vi "communicate.vi"(0 "Communication in":refnum<class "Communication.lvclass">, 1 "grSIM replacement":cluster{"robots":T4[], "ball":T5}, 2 "replace active":bool, 5 "Game":refnum<class "Game.lvclass">, 7 "Com UDP":T3={"UDP GrSim TX"=TRUE, "Address:"="127.0.0.1", "Port:"=20011}, 9 "Com Serial":T2, 11 "error in (no error)":errorcluster, 12 "Com SOS":T1={"UDP SOS TX "=FALSE, "SOS Port: 2"=10025, "SOS Port: "=10021, "SOS Address:"="192.168.0.101"}, 13 "FIRASim?":bool=TRUE) -> (4 "Communication out":refnum<class "Communication.lvclass">, 6 "Comm TX FPS":dbl, 10 "AllyRef":refnum<class "Ally.lvclass">, 15 "error out":errorcluster)   [LabVIEW 2023, in "Communication.lvclass"]
uses:
  Communication.lvclass
  Paths/grSim Packet Command UDP Test Folder/grSim/grSim RobotReplacement.ctl
  Paths/grSim Packet Command UDP Test Folder/grSim/grSim_BallReplacement.ctl
  Vision_class/Old vision/SSL Detection Frame Simple Estimator Cameras VelCmd Folder/Core/AI Input.ctl
  Vision_class/Old vision/Controls/AI Robot.ctl
  Vision_class/Old vision/Controls/Functions Enum.ctl
  Vision_class/Old vision/Controls/AttackerStates.ctl
  Vision_class/Old vision/Controls/PathDests.ctl
  Vision_class/Old vision/Controls/PathDest.ctl
  Game_class/Navigation/VSSNavigation/VSSAttackerStates.ctl
  Vision_class/Old vision/SSL Detection Frame Simple Estimator Cameras VelCmd Folder/Core/AI Ball.ctl
  Vision_class/Old vision/SSL Detection Frame Simple Estimator Cameras VelCmd Folder/Core/Field Size.ctl
  Vision_class/Old vision/SSL Detection Frame Simple Estimator Cameras VelCmd Folder/Core/AI Judge.ctl
  Paths/MessageAI_State Folder/Intel/Command Enum.ctl
  Vision_class/Old vision/SSL Detection Frame Simple Estimator Cameras VelCmd Folder/Util/Events/Events.ctl
  Game_class/Game.lvclass
  Controls/ComUDP.ctl
  Controls/ComSerial.ctl
  Controls/ComSOS.ctl
  Ally_class/Ally.lvclass
panel:
  in  "IA States":T6={"our_robots"=[], "enemy_robots"=[], "balls"=[], "geometry"={"line_width"=0, "field_length"=0, "field_width"=0, "boundary_width"=0, "referee_width"=0, "goal_width"=0, "goal_depth"=0, "goal_wall_width"=0, "center_circle_radius"=0, "defense_radius"=0, "defense_stretch"=0, "free_kick_from_defense_dist"=0, "penalty_spot_from_field_line_dist"=0, "penalty_line_from_spot_dist"=0}, "IA Judge"={"stage"="", "command"="", "our_goalie_id"=0.0, "enemy_goalie_id"=0.0, "command enum"=enum."Halt", "Time"=enum."Azul"}, "Received Timestamp"=timestamp(0 s since 1904-01-01), "Events"={"Touch"=FALSE, "Ball out"=FALSE, "id touch"=0.0, "Ball out of \nVision"=FALSE, "Ball inside \nGoalie area"=FALSE, "Robot not responding"=FALSE, "Robots responding status"=[1.0, 1.0, 1.0, 1.0, 1.0, 1.0], "Enemy Ball \nPossession"=FALSE, "Pass State"=FALSE, "id end of pass"=0.0, "Kick"=FALSE, "Id ini Possession"=0.0, "Ball Possesion"=FALSE, "Id Possesion"=0.0, "Direct Kick"=FALSE, "2nd Strk Ativo"=FALSE}}
  out "grSim":cluster{"robots":T4[], "ball":T5}
  out "Total Delay":dbl format="%#.5g"
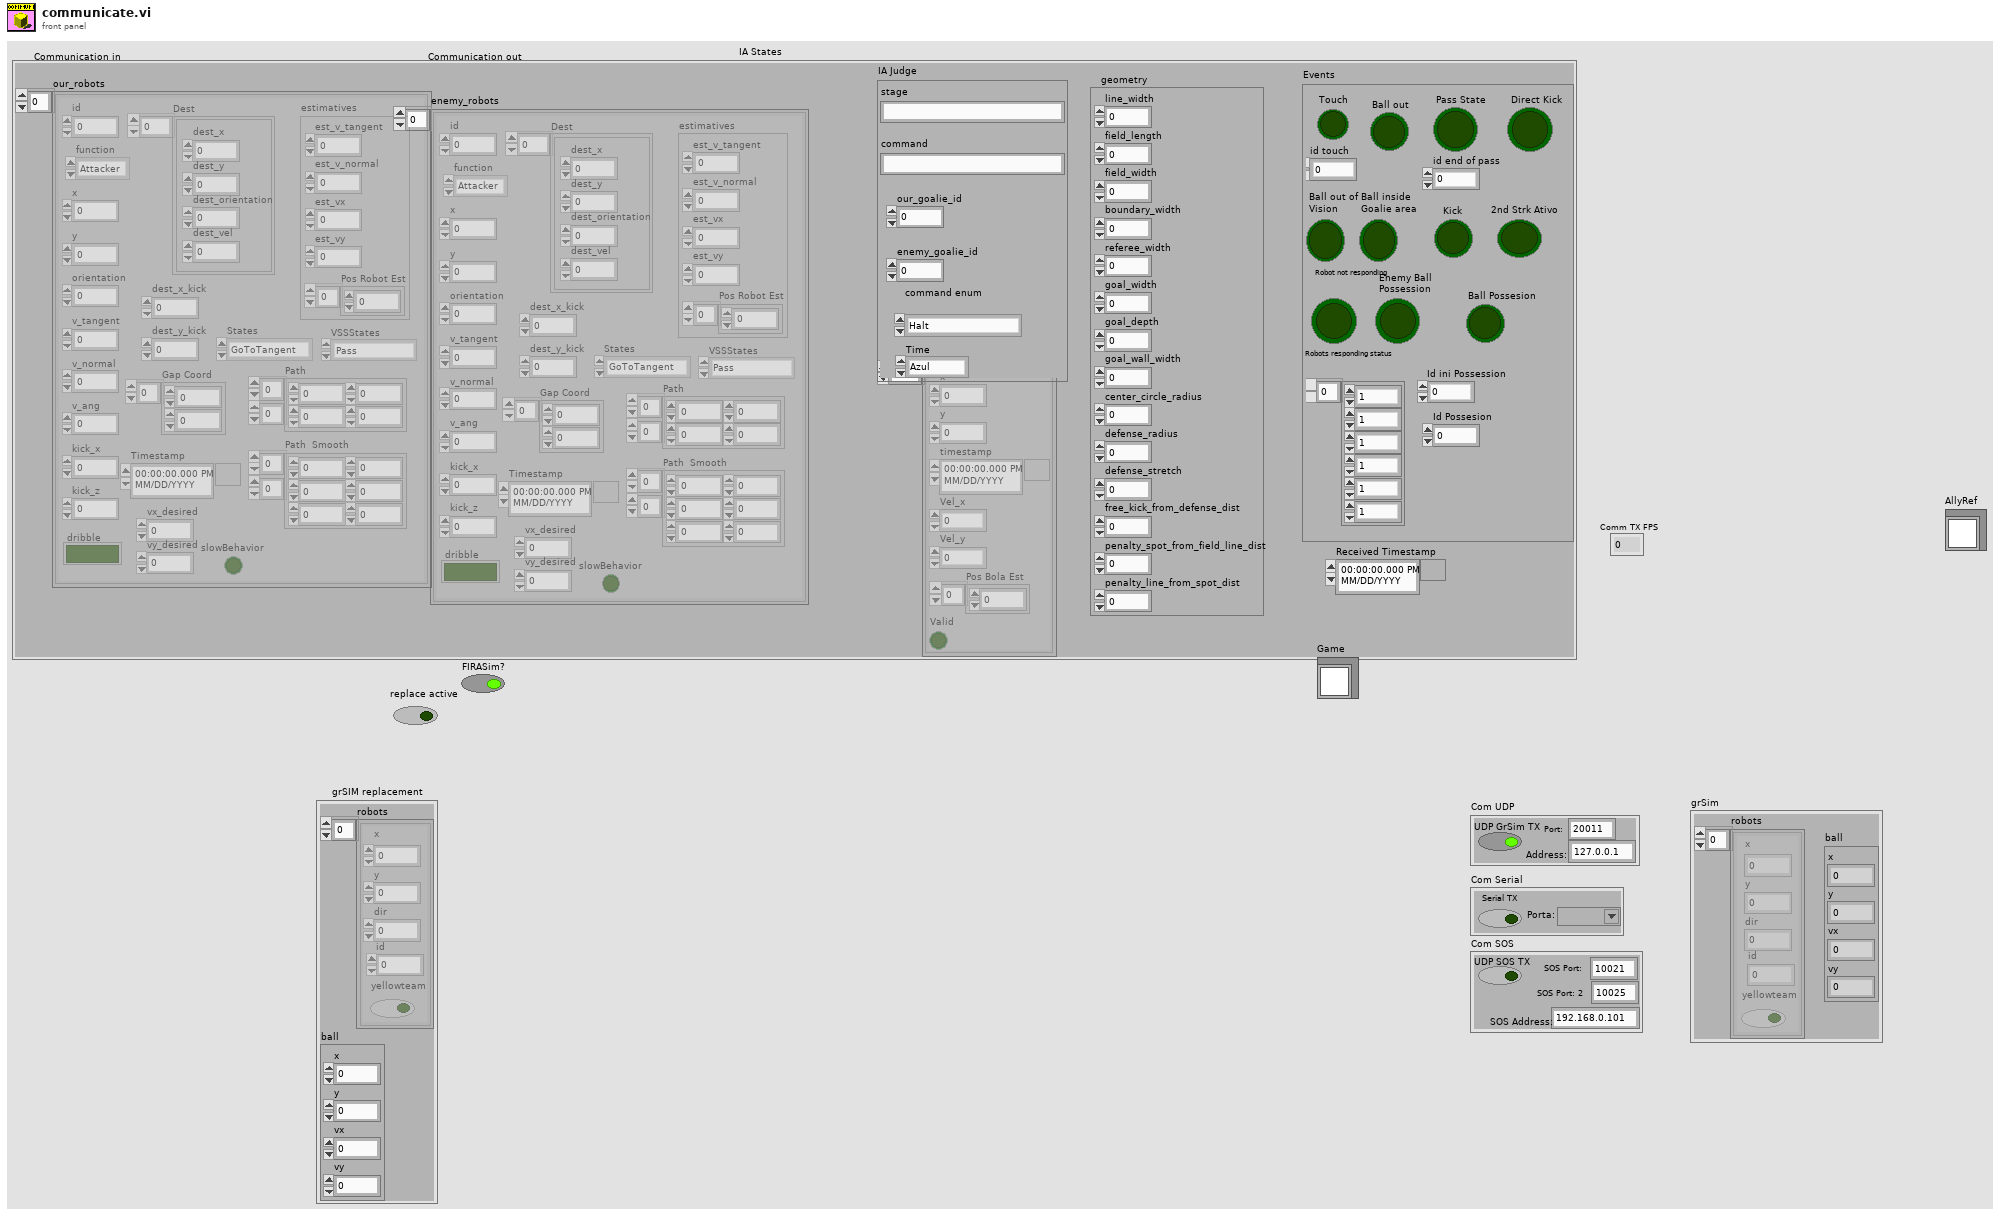
[diagram p1: front panel]
types:
  T1 = typedef "ComSOS.ctl" = cluster{"UDP SOS TX ":bool, "SOS Port: 2":u16, "SOS Port: ":u16, "SOS Address:":string}
  T2 = typedef "ComSerial.ctl" = cluster{"Serial TX":bool, "Porta:":refnum<visa-resource-name>}
  T3 = typedef "ComUDP.ctl" = cluster{"UDP GrSim TX":bool, "Address:":string, "Port:":u16}
  T4 = typedef "grSim RobotReplacement.ctl" = cluster{"x":dbl, "y":dbl, "dir":dbl, "yellowteam":bool, "id":u32}
  T5 = typedef "grSim_BallReplacement.ctl" = cluster{"x":dbl, "y":dbl, "vx":dbl, "vy":dbl}
  T6 = typedef "AI Input.ctl" = cluster{"our_robots":T7[], "enemy_robots":T7[], "balls":T13[], "geometry":T14, "IA Judge":T15, "Received Timestamp":timestamp, "Events":T17}
  T7 = typedef "AI Robot.ctl" = cluster{"id":u32, "function":T8, "x":dbl, "y":dbl, "orientation":dbl, "v_tangent":dbl, "v_normal":dbl, "v_ang":dbl, "kick_x":dbl, "kick_z":dbl, "dribble":bool, "Timestamp":timestamp, "estimatives":cluster{"est_v_tangent":dbl, "est_v_normal":dbl, "est_vx":dbl, "est_vy":dbl, "Pos Robot Est":dbl[]}, "dest_x_kick":dbl, "dest_y_kick":dbl, "Gap Coord":dbl[], "States":T9, "Path ":dbl[][], "Path  Smooth":dbl[][], "Dest":T10, "vx_desired":dbl, "vy_desired":dbl, "slowBehavior":bool, "VSSStates":T12}
  T8 = typedef "Functions Enum.ctl" = enum16{"2nd Striker", "Attacker", "Goalie", "Defender", "Striker", "Goto 0", "Dummy", "Kicker", "ZigZag 0", "ZigZag 1", "ZigZag 2", "ZigZag 3", "ZigZag 4", "ZigZag 5", "ZigZag 6", "ZigZag 7", "ZigZag 8", ""}
  T9 = typedef "AttackerStates.ctl" = enum16{"Pass", "GoToTangent", "BallGetting", "GoToKick", ""}
  T10 = typedef "PathDests.ctl" = T11[]
  T11 = typedef "PathDest.ctl" = cluster{"dest_x":dbl, "dest_y":dbl, "dest_orientation":dbl, "dest_vel":dbl}
  T12 = typedef "VSSAttackerStates.ctl" = enum16{"Pass", "GoToTangent", "BallGetting", "GoToKick", "Rotate anti-clockwise", "Rotate Clockwise", ""}
  T13 = typedef "AI Ball.ctl" = cluster{"x":dbl, "y":dbl, "timestamp":timestamp, "Vel_x":dbl, "Vel_y":dbl, "Pos Bola Est":dbl[], "Valid":bool}
  T14 = typedef "Field Size.ctl" = cluster{"line_width":u32, "field_length":u32, "field_width":u32, "boundary_width":u32, "referee_width":u32, "goal_width":u32, "goal_depth":u32, "goal_wall_width":u32, "center_circle_radius":u32, "defense_radius":u32, "defense_stretch":u32, "free_kick_from_defense_dist":u32, "penalty_spot_from_field_line_dist":u32, "penalty_line_from_spot_dist":u32}
  T15 = typedef "AI Judge.ctl" = cluster{"stage":string, "command":string, "our_goalie_id":dbl, "enemy_goalie_id":dbl, "command enum":T16, "Time":enum16{"Azul", "Amarelo"}}
  T16 = typedef "Command Enum.ctl" = enum16{"Halt", "Stop", "Force Start", "PKA Normal Start", "Prepare Kickoff Ally", "PKE Normal Start", "Prepare Kickoff Enemy", "Prepare Penalty Ally", "PPA Normal Start", "Prepare Penalty Enemy", "PPE Normal Start", "Direct Free Enemy", "Direct Free Ally", "Indirect Free Enemy", "Indirect Free Ally", "Timeout Enemy", "Timeout Ally", "Goal Enemy", "Goal Ally", "Ball Placement Enemy", "Ball Placement Ally", "Normal Half Time", "Extra Time Break", "Extra Half Time", "None", "Post Game"}
  T17 = typedef "Events.ctl" = cluster{"Touch":bool, "Ball out":bool, "id touch":dbl, "Ball out of \nVision":bool, "Ball inside \nGoalie area":bool, "Robot not responding":bool, "Robots responding status":dbl[], "Enemy Ball \nPossession":bool, "Pass State":bool, "id end of pass":dbl, "Kick":bool, "Id ini Possession":dbl, "Ball Possesion":bool, "Id Possesion":dbl, "Direct Kick":bool, "2nd Strk Ativo":bool}
  T18 = typedef "grSim Robot Command.ctl" = cluster{"id":u32, "kickspeedx":sgl, "kickspeedz":sgl, "veltangent":sgl, "velnormal":sgl, "velangular":sgl, "spinner":bool, "wheelspeed":bool, "wheel1":sgl, "wheel2":sgl, "wheel3":sgl, "wheel4":sgl}
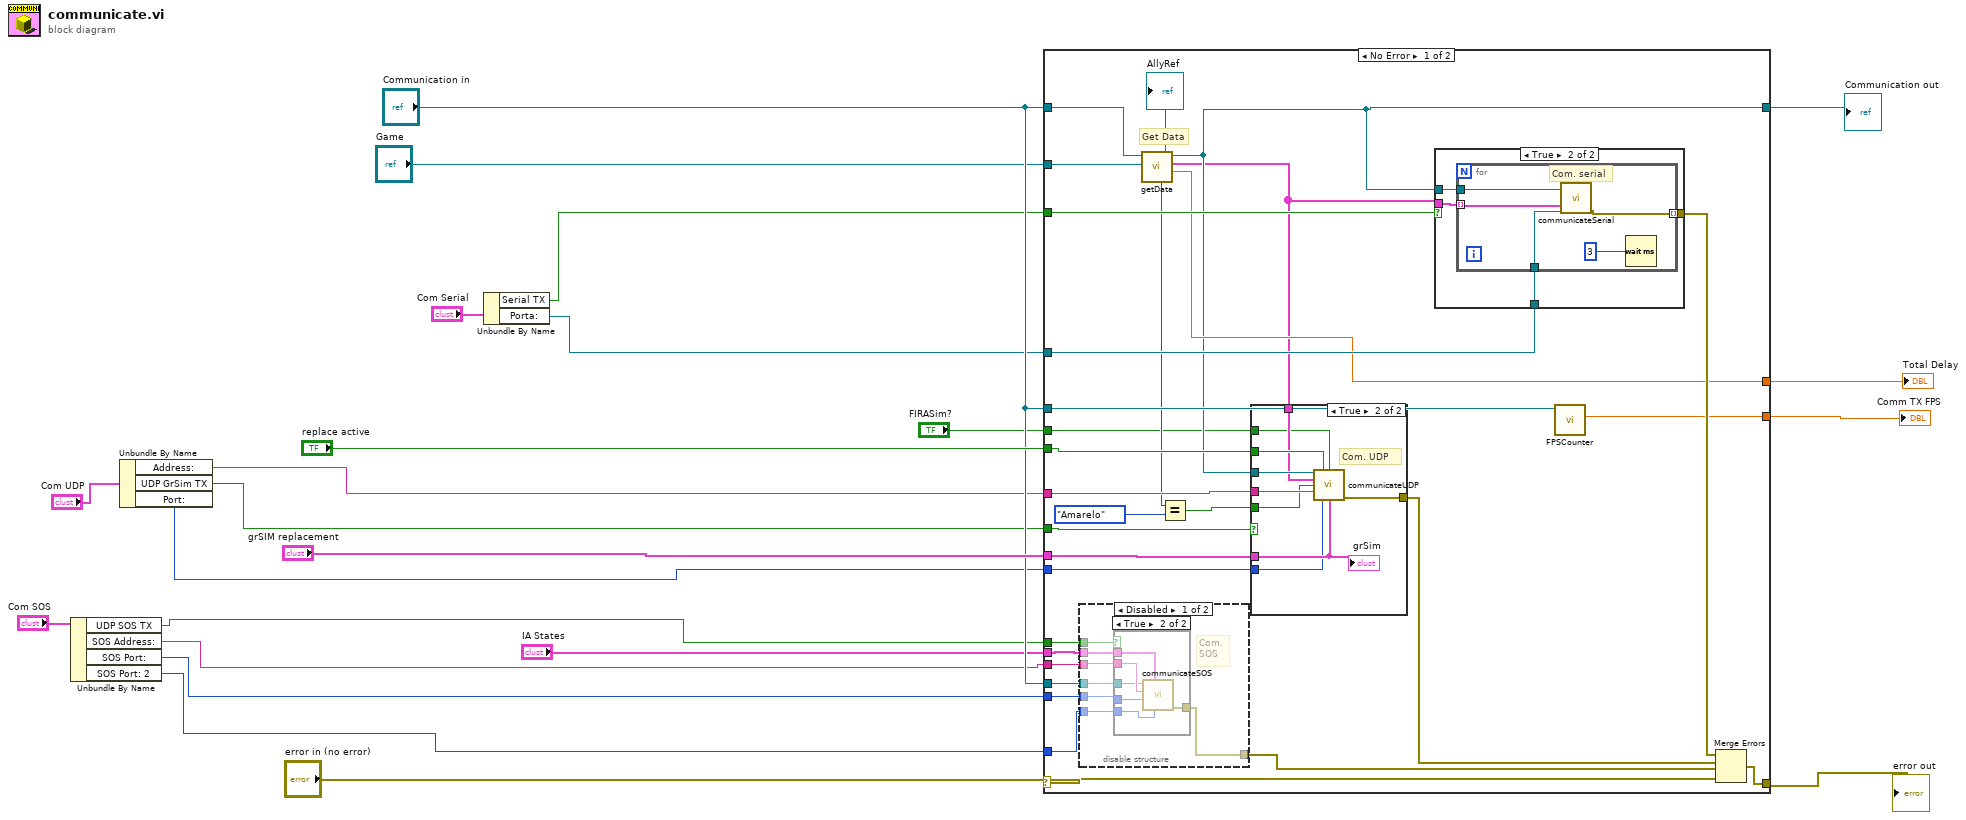
[diagram p0: block diagram]
diagram:
  n1 = Unbundle By Name("Com SOS") -> ("UDP SOS TX"=w8:bool, "SOS Address:"=w7:string, "SOS Port:"=w6:u16, "SOS Port: 2"=w5:u16)
  n2 = Unbundle By Name("Com UDP") -> ("Address:"=w12:string, "UDP GrSim TX"=w11:bool, "Port:"=w10:u16)
  n3 = Unbundle By Name("Com Serial") -> ("Serial TX"=w2:bool, "Porta:"=w3:refnum<visa-resource-name>)
  n4 = case shown="No Error" "error in (no error)" {
    selector: "error in (no error)" -> [w39 w86]
    tunnel: [w40 w86] -> w19
    tunnel: [w29 w85] -> w22
    tunnel: "Communication in" -> [w30 w85]
    tunnel: "IA States" -> [w50 _]
    tunnel: "grSIM replacement" -> [w52 _]
    tunnel: "replace active" -> [w47 _]
    tunnel: w11 -> [w51 _]
    tunnel: w10 -> [w49 _]
    tunnel: w12 -> [w48 _]
    tunnel: w8 -> [w46 _]
    tunnel: w6 -> [w45 _]
    tunnel: w5 -> [w44 _]
    tunnel: w7 -> [w43 _]
    tunnel: w2 -> [w42 _]
    tunnel: w3 -> [w41 _]
    tunnel: "Communication in" -> [w36 _]
    tunnel: "Communication in" -> [w35 _]
    tunnel: [w33 _] -> w17
    tunnel: [w31 _] -> w16
    tunnel: "Game" -> [w27 _]
    tunnel: "FIRASim?" -> [w24 _]
    frame No Error {
      # "Get Data"
      n5 = disable-structure shown="Disabled" {
        disable-tunnel: w50 -> [w60 _]
        disable-tunnel: w46 -> [w59 _]
        disable-tunnel: w45 -> [w58 _]
        disable-tunnel: w44 -> [w57 _]
        disable-tunnel: w43 -> [w56 _]
        disable-tunnel: [w55 _] -> w38
        disable-tunnel: w36 -> [w54 _]
        frame Disabled {
          # "Com.\nSOS"
          n6 = case shown="True" w59 {
            tunnel: w60 -> [_ w66]
            tunnel: w58 -> [_ w64]
            tunnel: w57 -> [_ w63]
            tunnel: w56 -> [_ w65]
            tunnel: [_ w62] -> w55
            tunnel: w54 -> [_ w61]
            frame False {
            }
            frame True {
              n7 = call-dynamic "communicateSOS.vi"("SOS Port: 2"=w63, "AI State"=w66, "SOS Port:"=w64, "SOS Address:"=w65, "Communication in"=w61) -> ("error out"=w62:errorcluster)  [unwired: 5 in, 1 out]
            }
          }
        }
        frame Enabled {
        }
      }
      n8 = call-dynamic "getData.vi"("Game"=w27, "Communication in"=w30) -> ("Total Delay"=w31:dbl, "Robot Data"=w26:T18[], "Communication out"=w29:refnum<class "Communication.lvclass">, "Team Color"=w28:enum16{"Azul", "Amarelo"}, "AllyRef"=→"AllyRef":refnum<class "Ally.lvclass">)  [unwired: 4 in, 1 out]
      n9 = Equal?(x=w28, y=enum16{"Azul", "Amarelo"}."Amarelo") -> (x = y?=w53:bool)
      n10 = case shown="True" w51 {
        tunnel: w53 -> [_ w80]
        tunnel: w47 -> [_ w79]
        tunnel: w52 -> [_ w84]
        tunnel: w49 -> [_ w83]
        tunnel: w48 -> [_ w81]
        tunnel: [_ w82] -> w37
        tunnel: w29 -> [_ w78]
        tunnel: w26 -> [_ w77]
        tunnel: w24 -> [_ w76]
        frame False {
        }
        frame True {
          # "Com. UDP"
          n11 = call-dynamic "communicateUDP.vi"("Communication in"=w78, "Replace Now"=w79, "FIRASim?"=w76, "Robots"=w77, "isMyTeamYellow"=w80, "Address:"=w81, "Port:"=w83, "grSim replacement"=w84) -> ("error out"=w82:errorcluster)  [unwired: 6 in, 1 out]
          "grSim" <- w84
        }
      }
      n12 = case shown="True" w42 {
        tunnel: w26 -> [_ w70]
        tunnel: w41 -> [_ w69]
        tunnel: [_ w68] -> w34
        tunnel: w29 -> [_ w67]
        frame False {
        }
        frame True {
          n13 = for {
            tunnel: w70 -> [w74] mode=indexing
            tunnel: w69 -> [w73]
            tunnel: [w72] -> w68 mode=indexing
            tunnel: w67 -> [w71]
            # "Com. serial"
            n14 = call-dynamic "communicateSerial.vi"("Porta:"=w73, "Robots"=w74, "Communication in"=w71) -> ("error out"=w72:errorcluster)  [unwired: 7 in, 1 out]
            n15 = Wait (ms)(milliseconds to wait=u32 3) -> ()  [unwired: 1 out]
          }
        }
      }
      n16 = call-dynamic "FPSCounter.vi"("Communication in"=w35) -> ("Comm TX FPS"=w33:dbl)  [unwired: 8 in, 2 out]
      n17 = Merge Errors(w34, w37, w38, w39) -> (w40:errorcluster)
    }
    frame Error {
    }
  }
  "error out" <- w19
  "Communication out" <- w22
  "Comm TX FPS" <- w17
  "Total Delay" <- w16
